vi "LIN_demo.vi"() -> ()   [LabVIEW 2020, in "zlgcan.lvlib"]
uses:
  zlgcan.lvlib
  ZCAN_LIN_MSG.ctl
  ZCAN_LIN_INIT_CONFIG_USBCANFD.ctl
  ZCAN_LIN_SUBSCIBE_CFG.ctl
  ZCAN_LIN_PUBLISH_CFG.ctl
  bin/zlgcan_wrap_LIN.dll
panel:
  in  "开启LIN":bool
  in  "?":T1(tab)
  in  "索引":u32(ring) items=["0", "1", "2", "3", "4", "5", "6", "7", "8"]
  in  "CAN卡型号":u32(ring)=41 items=["USBCANFD-400U"=76, "USBCANFD-800U"=59, "USBCANFD-200U"=41, "USBCANFD-100U"=42, "USBCANFD-MINI"=43]
  in  "LIN波特率（取值 1000~20000）":u32(ring)=9600 items=["19200"=19200, "9600"=9600, "4800"=4800, "2400"=2400]
  out "通道索引":u32(ring) items=["1"=1, "0"=0]
  in  "校验方式 （1-经典校验 2-增强校验 3-自动(即经典校验跟增强校验都会进行轮询)）":u8(ring)=1 items=["3"=3, "2"=2, "1"=1]
  out "LIN工作模式（从站为0，主站为1）":u8(ring) items=["1"=1, "0"=0]
  out "Device_handle(out)":u32
  out "lin1_index_handle(out)":u32
  out "lin0_index_handle(out)":u32
  in  "ID(hex)":u8=1 format="%x"
  in  "datalen":u8=8
  in  "数组长度":u32=1
  in  "chksumMode":u8=1
  in  "设置发布":bool
  in  "data十六进制hex":T2={"data[0]"=1, "data[1]"=2, "data[2]"=3, "data[3]"=4, "data[4]"=5, "data[5] "=6, "data[6] "=7, "data[7] "=8} {"data[7]" format="%x"; "data[6]" format="%x"; "data[5]" format="%x"; "data[0]" format="%x"; "data[1]" format="%x"; "data[2]" format="%x"; "data[3]" format="%x"; "data[4]" format="%x"}
  in  "设置订阅":bool
  in  "ID(Hex)":u8=1 format="%x"
  in  "datalen":u8=8
  in  "chkSumMode":u8=1
  in  "数组长度":u32=1
  in  "chnl 主站1":u8=1
  in  "dataType\n0为LIN数据":u8
  in  "ZCANLINData.PID(十六进制hex)":u8=1 format="%x"
  in  "datalen 数据长度":u8
  in  "timeStamp 时间戳 单位us":u64
  in  "dir 传输方向 0接收，1发送":u8
  in  "发送":bool
  out "已接收的帧数":u32
  out "LIN报文显示（仅显示LIN0从站的数据，方向针对的数据段而言）LIN类型为LIN错误数据则该数据出错，需要查看的话可自行二次开发":string[][](table)
  in  "LIN数据帧数组":T3[](array[typedef])
  in  "reserved":T4
  in  "ZCAN_LIN_PUBLISH_CFG":T5
  in  "reserved":T4
  in  "?":T6
  in  "chkSum 数据校验":u8
  in  "Reserved":u16
  in  "?":T7
  in  "ZCAN_LIN_MSG":T3
  in  "stop":bool
  in  "停止按钮":bool
  # "demo演示：LIN0通道做从站，LIN1通道做主站，仅主站可以往外发数据"
  # "流程：启动LIN----设置发布的ID等参数后，点击【设置发布】----LIN主站进行发送头部（PID跟发布的ID相同）"
  # "后面板已循环开启俩个LIN通道"
  # "1. 确保电脑有VC++ 2005/2008/2010/2013运行库（对应32，64位）,微软常用运行库合集，点击下载（35M）。\n    http://manual.zlg.cn/Public/Uploads/2020-06-05/5ed995c271414.zip"
  # "2，如果打开设备失败，可能原因：\n（1）已经打开过一次，没有正常关闭的情况下，继续点击“打开设备”，是无法打开的。\n     需要USB重新拔插，LABVIEW重启（全部关闭），然后再“打开设备”。\n (2) 项目路径不能有中文繁体。"
  # "LIN0(从站)设置发布，仅举例，可到后面板修改"
  # "用LIN1(主站)进行订阅数据"
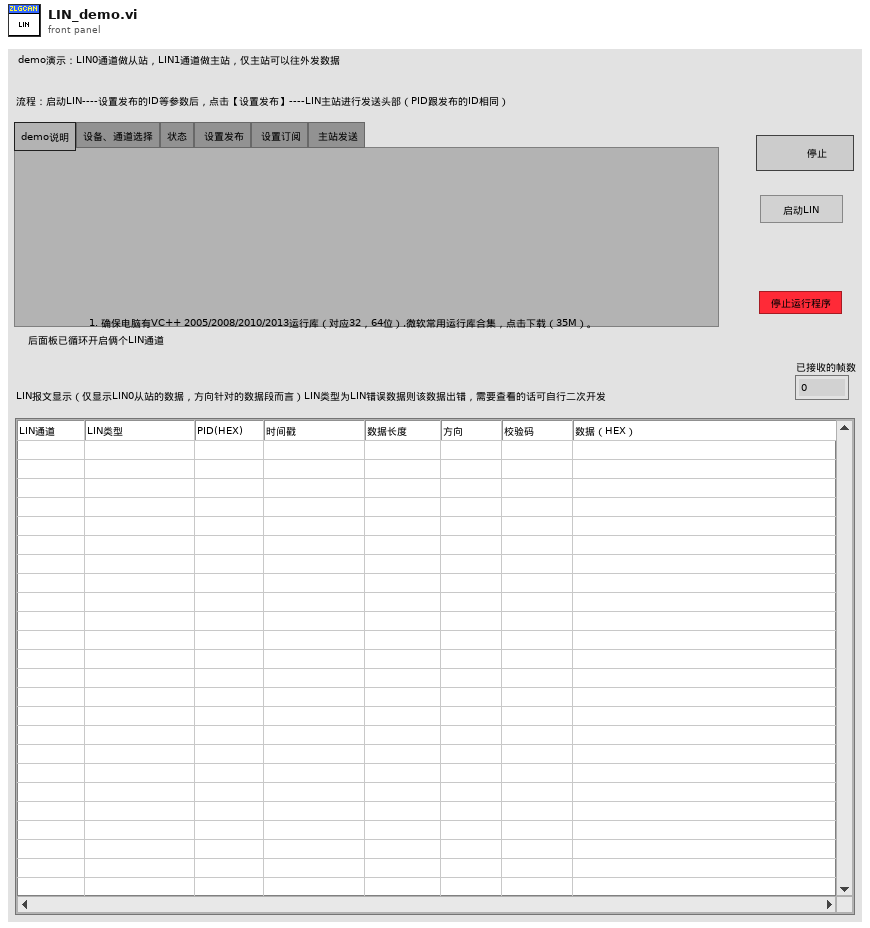
[diagram p1: front panel]
types:
  T1 = enum32{"demo说明", "设备、通道选择", "状态", " 设置发布", " 设置订阅", " 主站发送"}
  T2 = cluster{"data[0]":u8, "data[1]":u8, "data[2]":u8, "data[3]":u8, "data[4]":u8, "data[5] ":u8, "data[6] ":u8, "data[7] ":u8}
  T3 = typedef "zlgcan.lvlib/ZCAN_LIN_MSG.ctl" = cluster{"chnl":u8, "dataType":u8, "reserved 0":cluster{"CAN数据[0]":u8, "CAN数据[1]":u8, "CAN数据[2]":u8, "CAN数据[3]":u8, "CAN数据[4]":u8, "CAN数据[5]":u8}, "ZCANLINData":cluster{"PID":u8, "reserved":cluster{"CAN数据[0]":u8, "CAN数据[1]":u8, "CAN数据[2]":u8, "CAN数据[3]":u8, "CAN数据[4]":u8, "CAN数据[5]":u8, "CAN数据[6]":u8}, "RxData":cluster{"timeStamp":u64, "datalen":u8, "dir":u8, "chkSum":u8, "reserved[0]":u8, "reserved[1]":u8, "reserved[2] ":u8, "reserved[3]":u8, "reserved[4]":u8, "reserved[5]":u8, "reserved[6] ":u8, "reserved[7] ":u8, "reserved[8]":u8, "reserved[9] ":u8, "reserved[10] ":u8, "reserved[11] ":u8, "reserved[12] ":u8, "data[0]":u8, "data[1]":u8, "data[2]":u8, "data[3]":u8, "data[4]":u8, "data[5]":u8, "data[6]":u8, "data[7]":u8}}, "reserved 1":cluster{"CAN数据[0]":u8, "CAN数据[1]":u8, "CAN数据[2]":u8, "CAN数据[3]":u8, "CAN数据[4]":u8, "CAN数据[5]":u8}}
  T4 = cluster{"reserved[0]":u8, "reserved[1]":u8, "reserved[2]":u8, "reserved[3]":u8, "reserved[4]":u8}
  T5 = typedef "zlgcan.lvlib/ZCAN_LIN_PUBLISH_CFG.ctl" = cluster{"ID":u8, "datalen":u8, "data":cluster{"data[0]":u8, "data[1]":u8, "data[2]":u8, "data[3]":u8, "data[4]":u8, "data[5] ":u8, "data[6] ":u8, "data[7] ":u8}, "chkSumMode":u8, "reserved":cluster{"reserved[0]":u8, "reserved[1]":u8, "reserved[2]":u8, "reserved[3]":u8, "reserved[4]":u8}}
  T6 = typedef "zlgcan.lvlib/ZCAN_LIN_SUBSCIBE_CFG.ctl" = cluster{"ID":u8, "datalen":u8, "chkSumMode":u8, "reserved":cluster{"reserved[0]":u8, "reserved[1]":u8, "reserved[2]":u8, "reserved[3]":u8, "reserved[4]":u8}}
  T7 = typedef "zlgcan.lvlib/ZCAN_LIN_INIT_CONFIG_USBCANFD.ctl" = cluster{"LinMode":u8, "chkSumMode":u8, "Reserved":u16, "linBaud":u32}
  T8 = cluster{"CAN数据[0]":u8, "CAN数据[1]":u8, "CAN数据[2]":u8, "CAN数据[3]":u8, "CAN数据[4]":u8, "CAN数据[5]":u8}
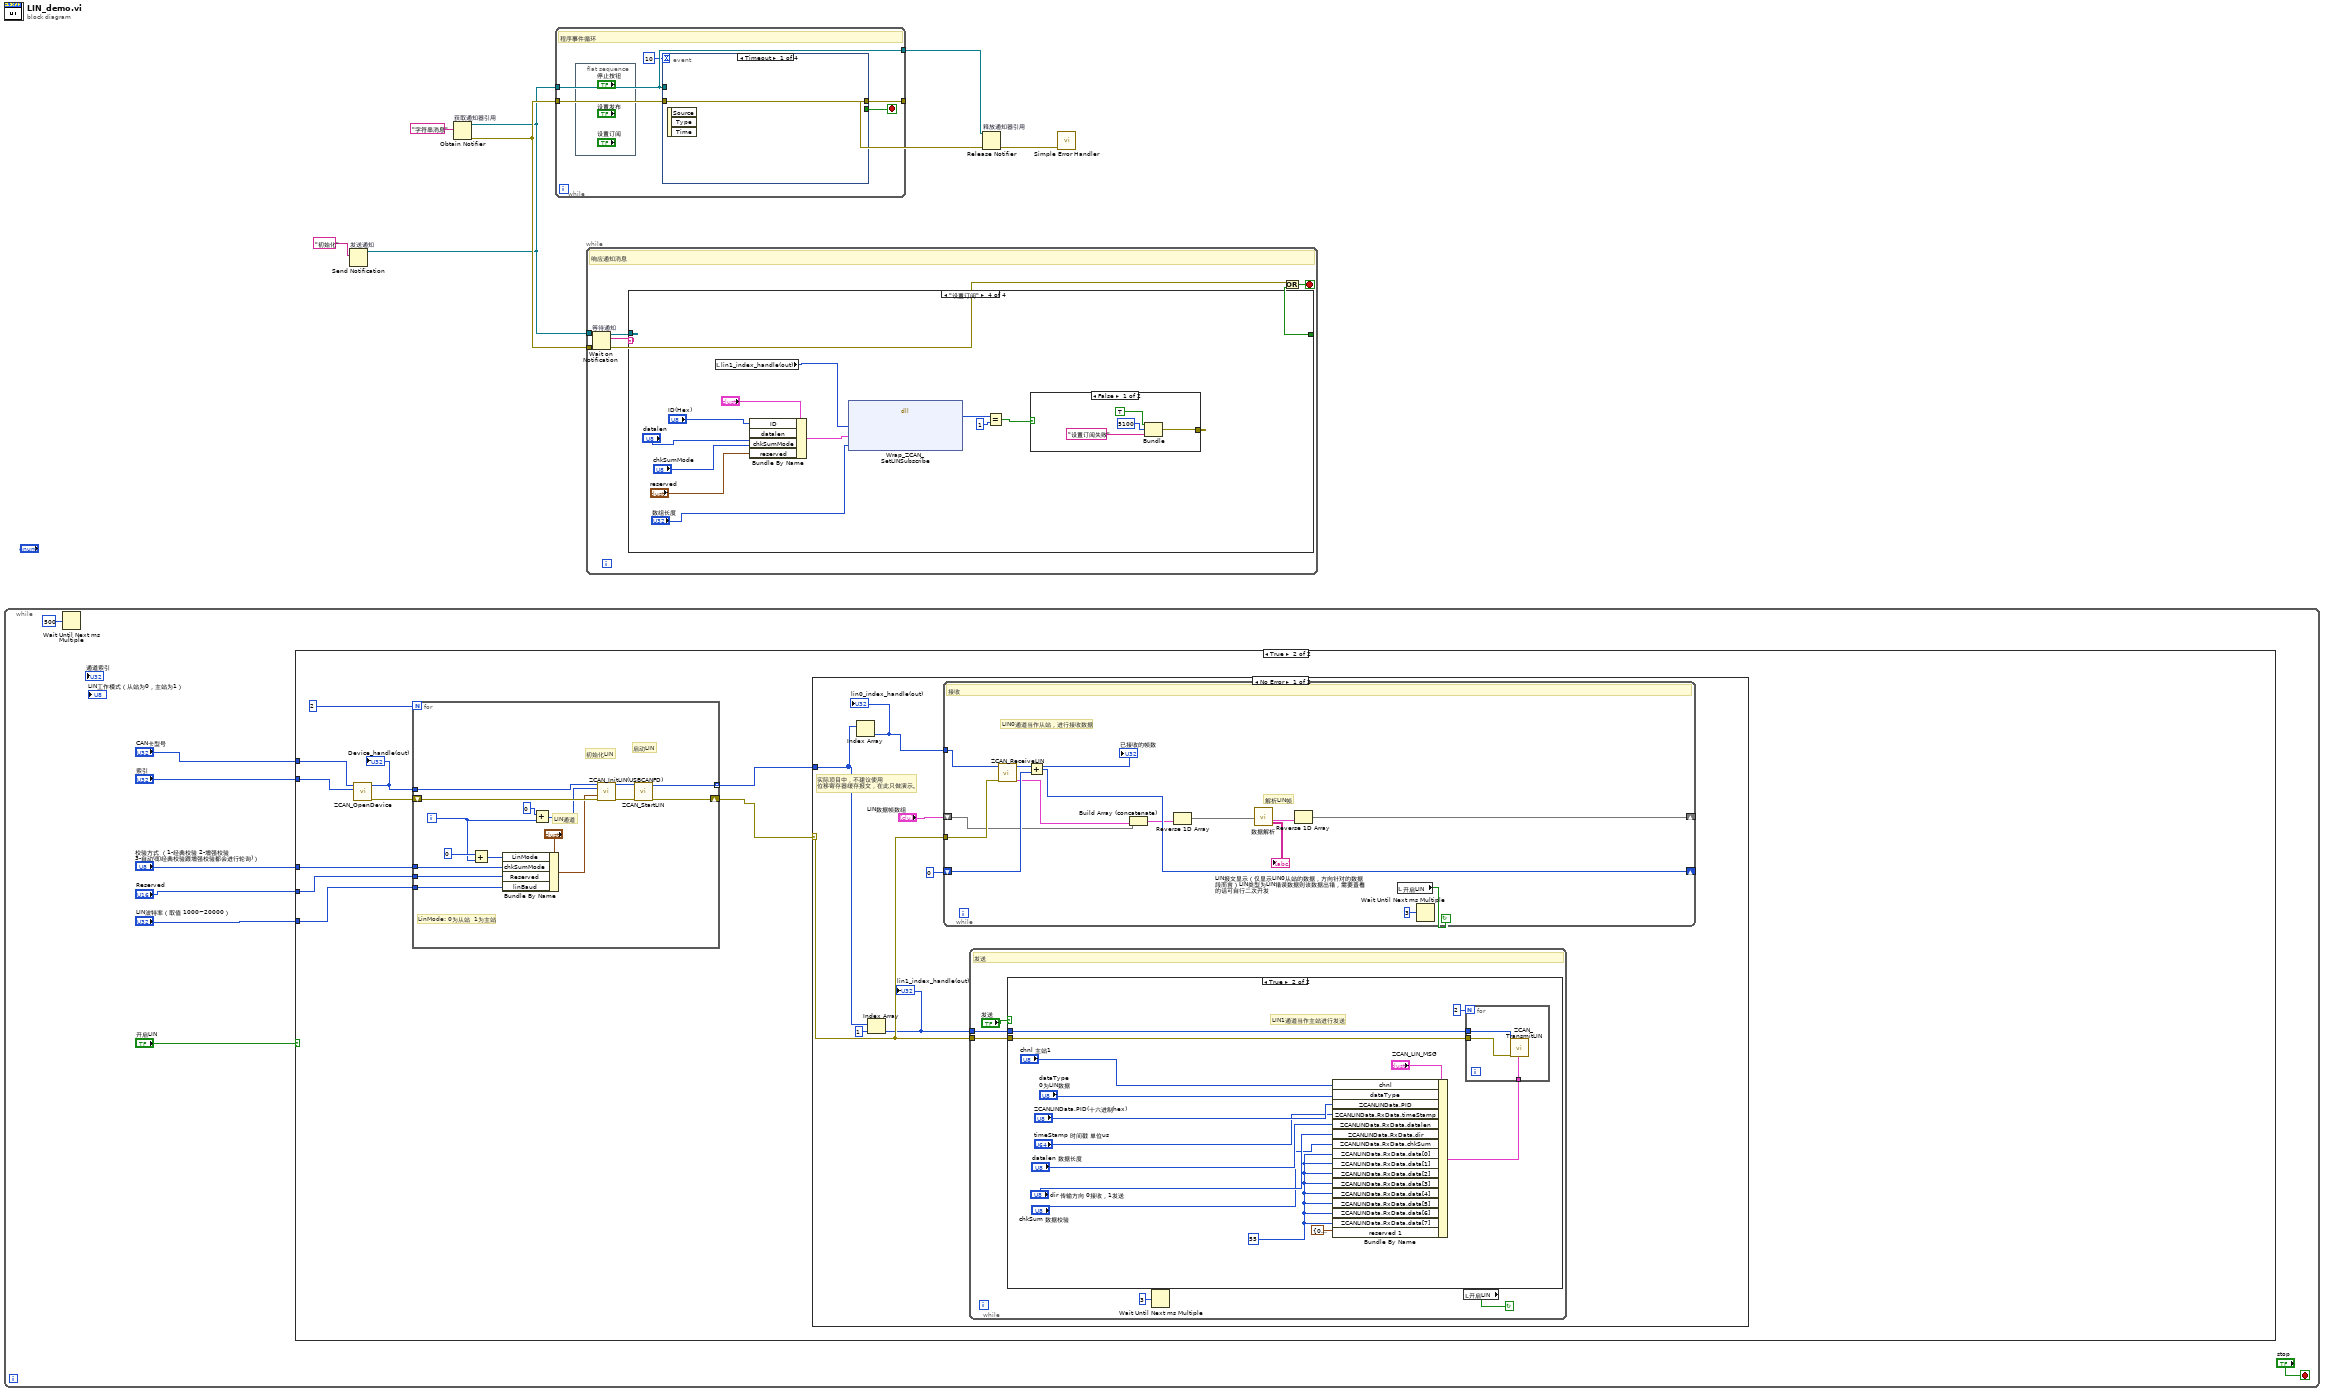
[diagram p0: block diagram]
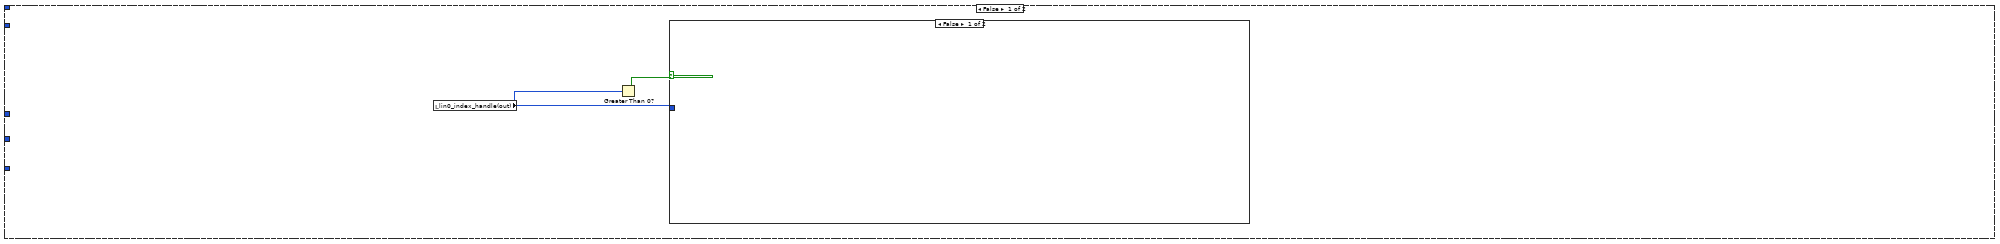
[diagram p2: hidden frame]
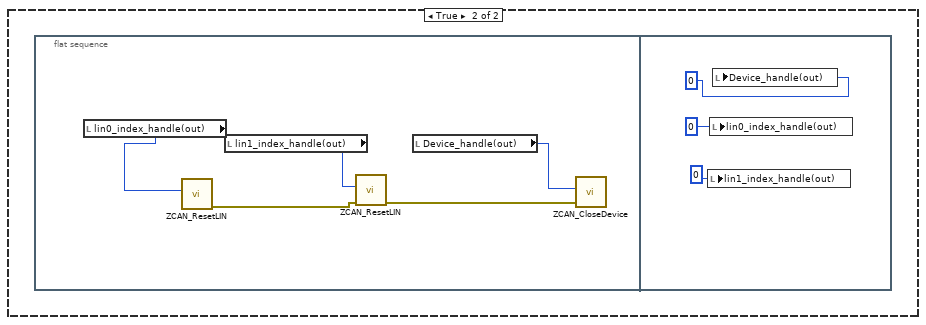
[diagram p3: hidden frame]
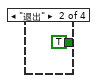
[diagram p7: hidden frame]
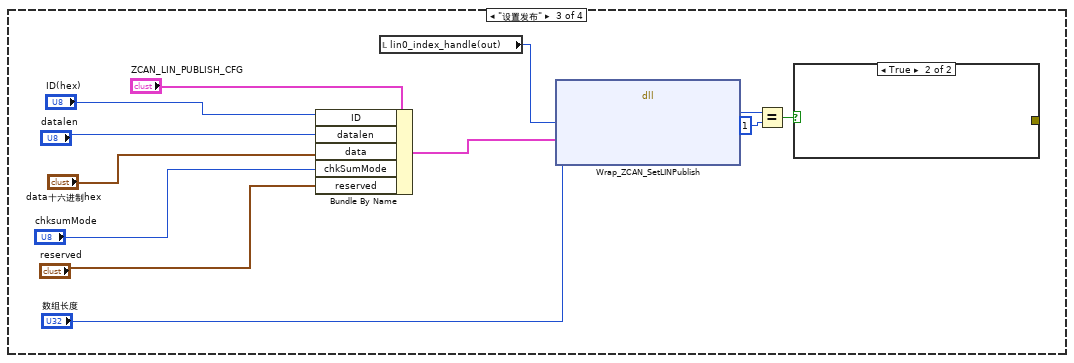
[diagram p8: hidden frame]
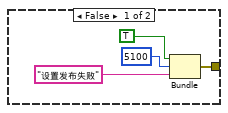
[diagram p9: hidden frame]
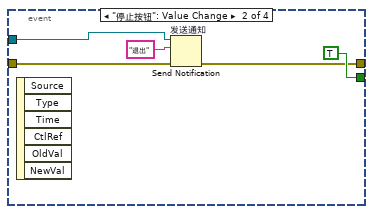
[diagram p11: hidden frame]
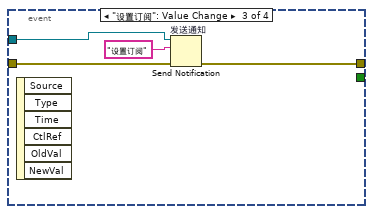
[diagram p12: hidden frame]
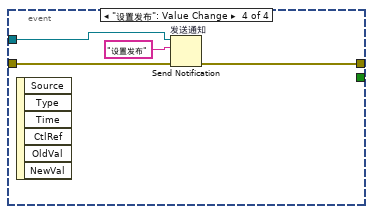
[diagram p13: hidden frame]
diagram:
  n1 = while {
    stop <- "stop" stop-if-true
    n2 = Wait Until Next ms Multiple(millisecond multiple=u32 500) -> ()  [unwired: 1 out]
    n3 = case shown="True" "开启LIN" {
      tunnel: "CAN卡型号" -> [_ w27]
      tunnel: "索引" -> [_ w26]
      tunnel: "LIN波特率（取值 1000~20000）" -> [_ w34]
      tunnel: "Reserved" -> [_ w33]
      tunnel: "校验方式 （1-经典校验 2-增强校验 3-自动(即经典校验跟增强校验都会进行轮询)）" -> [_ w31]
      frame False {
        # "关闭CAN卡"
        n4 = local read "lin0_index_handle(out)"() -> (w16:u32)
        n5 = Greater Than 0?(x=w16) -> (x > 0?=w17:bool)
        n6 = case shown="False" w17 {
          tunnel: w16 -> [_ _]
          frame False {
          }
          frame True {
            n7 = flat-sequence {
              frame #0 {
                n8 = local read "lin0_index_handle(out)"() -> (w22:u32)
                n9 = call "ZCAN_ResetLIN.vi"("lin_handle"=w22) -> ("error out"=w18:errorcluster)  [unwired: 9 in, 1 out]
                n10 = local read "lin1_index_handle(out)"() -> (w21:u32)
                n11 = call "ZCAN_ResetLIN.vi"("error in (no error)"=w18, "lin_handle"=w21) -> ("error out"=w20:errorcluster)  [unwired: 8 in, 1 out]
                n12 = local read "Device_handle(out)"() -> (w19:u32)
                n13 = call "ZCAN_CloseDevice.vi"("error in (no error)"=w20, "device_handle"=w19) -> ()  [unwired: 8 in, 2 out]
              }
              frame #1 {
                n14 = local write "lin1_index_handle(out)"(u32 0 ("lin1_index_handle(out)")) -> ()
                n15 = local write "lin0_index_handle(out)"(u32 0 ("lin0_index_handle(out)")) -> ()
                n16 = local write "Device_handle(out)"(u32 0 ("Device_handle(out)")) -> ()
              }
            }
          }
        }
      }
      frame True {
        n17 = call "ZCAN_OpenDevice.vi"("device_index"=w26, "device_type"=w27) -> ("error out"=w28:errorcluster, "DEVICE_HANDLE"=w29:u32)  [unwired: 6 in, 2 out]
        "Device_handle(out)" <- w29
        n18 = for {
          N: 2 -> [_]
          tunnel: [w36] -> w32 mode=indexing
          tunnel: w29 -> [w50]
          tunnel: w34 -> [w46]
          tunnel: w33 -> [w45]
          shift-right: [w49] -> w35
          shift-left: w28 -> [w51]
          tunnel: w31 -> [w39]
          i -> [w40]
          # "LinMode: 0为从站  1为主站"
          # "LIN通道"
          # "启动LIN"
          # "初始化LIN"
          n19 = Add(x=0, y=w40) -> (x+y=w41:i32)
          n20 = Bundle By Name(cluster="?", "LinMode"=w41, "chkSumMode"=w39, "Reserved"=w45, "linBaud"=w46) -> (w38:T7)
          n21 = Add(x=0, y=w40) -> (x+y=w44:i32)
          n22 = call "ZCAN_InitLIN(USBCANFD).vi"("device_hande"=w50, "lin_index"=w44, "ZCAN_LIN_INIT_CONFIG_USBCANFD"=w38, "error in (no error)"=w51) -> ("LIN_index_handle"=w37:u32, "error out"=w48:errorcluster)  [unwired: 10 in]
          n23 = call "ZCAN_StartLIN.vi"("error in (no error)"=w48, "lin_index_handle"=w37) -> ("error out"=w49:errorcluster, "lin_index_handle(out)"=w36:u32)  [unwired: 7 in, 1 out]
        }
        n24 = case shown="No Error" w35 {
          selector: w35 -> [w57 _]
          tunnel: w32 -> [w54 _]
          frame No Error {
            # "实际项目中，不建议使用\n位移寄存器缓存报文，在此只做演示。"
            n25 = Index Array(array=w54) -> (element=w53:u32)  [unwired: 1 in]
            "lin0_index_handle(out)" <- w53
            n26 = Index Array(array=w54, index=1 ("索引")) -> (element=w56:u32)
            "lin1_index_handle(out)" <- w56
            n27 = while {
              tunnel: w57 -> [w70]
              shift-right: [w71] -> _
              shift-left: 0 -> [w68]
              tunnel: w53 -> [w59]
              shift-right: [w60] -> _
              shift-left: "LIN数据帧数组" -> [w67]
              stop <- w69 continue-if-true
              # "解析LIN帧"
              # "LIN0通道当作从站，进行接收数据"
              # "接收"
              n28 = call "ZCAN_ReceiveLIN.vi"("error in (no error)"=w70, "channel_handle"=w59) -> ("LIN数据帧数组"=w62:T3[], "Receive_Num"=w66:u32)  [unwired: 4 in]
              "已接收的帧数" <- w66
              n29 = Add(x=w66, y=w68) -> (x+y=w71:u32)
              n30 = Build Array (concatenate)(w67, w62) -> (w65:T3[])
              n31 = Reverse 1D Array(array=w65) -> (reversed array=w64:T3[])
              n32 = call "数据解析.vi"("LIN数据帧数组"=w64) -> ("LIN数据帧数组 out"=w63:T3[], "LIN报文显示"=→"LIN报文显示（仅显示LIN0从站的数据，方向针对的数据段而言）LIN类型为LIN错误数据则该数据出错，需要查看的话可自行二次开发":string[][])  [unwired: 9 in]
              n33 = Reverse 1D Array(array=w63) -> (reversed array=w60:T3[])
              n34 = local read "开启LIN"() -> (w69:bool)
              n35 = Wait Until Next ms Multiple(millisecond multiple=u32 3) -> ()  [unwired: 1 out]
            }
            n36 = while {
              tunnel: w57 -> [w74]
              tunnel: w56 -> [w73]
              stop <- w75 continue-if-true
              # "发送"
              n37 = case shown="True" "发送" {
                tunnel: w74 -> [_ w89]
                tunnel: w73 -> [_ w90]
                frame False {
                }
                frame True {
                  w80 = u8 55 ("ZCANLINData.RxData.[data[0]")
                  # "LIN1通道当作主站进行发送"
                  n38 = Bundle By Name(cluster="ZCAN_LIN_MSG", "chnl"="chnl 主站1", "dataType"="dataType\n0为LIN数据", "ZCANLINData.PID"="ZCANLINData.PID(十六进制hex)", "ZCANLINData.RxData.timeStamp"="timeStamp 时间戳 单位us", "ZCANLINData.RxData.datalen"="datalen 数据长度", "ZCANLINData.RxData.dir"="dir 传输方向 0接收，1发送", "ZCANLINData.RxData.chkSum"="chkSum 数据校验", "ZCANLINData.RxData.data[0]"=w80, "ZCANLINData.RxData.data[1]"=w80, "ZCANLINData.RxData.data[2]"=w80, "ZCANLINData.RxData.data[3]"=w80, "ZCANLINData.RxData.data[4]"=w80, "ZCANLINData.RxData.data[5]"=w80, "ZCANLINData.RxData.data[6]"=w80, "ZCANLINData.RxData.data[7]"=w80, "reserved 1"=T8 {"CAN数据[0]"=0, "CAN数据[1]"=0, "CAN数据[2]"=0, "CAN数据[3]"=0, "CAN数据[4]"=0, "CAN数据[5]"=0}) -> (w88:T3)
                  n39 = for {
                    N: 2 -> [_]
                    tunnel: w90 -> [w94]
                    tunnel: w89 -> [w93]
                    tunnel: w88 -> [w92]
                    n40 = call "ZCAN_TransmitLIN.vi"("ZCAN_LIN_MSG"=w92, "error in (no error)"=w93, "lin_index_handle"=w94) -> ()  [unwired: 8 in, 1 out]
                  }
                }
              }
              n41 = Wait Until Next ms Multiple(millisecond multiple=u32 3) -> ()  [unwired: 1 out]
              n42 = local read "开启LIN"() -> (w75:bool)
            }
          }
          frame Error {
          }
        }
      }
    }
  }
  n43 = Obtain Notifier "获取通知器引用"(notification data type="字符串消息" ("元素数据类型")) -> (notifier out=w1:refnum<notifier>, error out=w6:errorcluster)  [unwired: 3 in, 1 out]
  n44 = Send Notification "发送通知"(notification="初始化" ("通知"), notifier=w1) -> ()  [unwired: 1 in, 2 out]
  n45 = while "While循环" {
    tunnel: w1 -> [w96]
    tunnel: [w96] -> w7
    tunnel: w6 -> [w98]
    tunnel: [w97] -> w5
    stop <- w99 stop-if-true
    # "程序事件循环"
    n46 = flat-sequence {
      frame #0 {
      }
    }
    n47 = event shown="[0] Timeout" {
      selector: _ -> [_ _ _ _]
      dyn-events: _ -> [_ _ _ _]
      timeout: 10 -> [_ _ _ _]
      tunnel: w96 -> [_ w103 w108 w112]
      tunnel: [_ TRUE _ _] -> w99
      tunnel: w98 -> [w100 w102 w107 w111]
      tunnel: [w100 w101 w106 w110] -> w97
      event Timeout {
        n48 = event-data() -> ()  [unwired: 1 in, 3 out]
      }
      event "停止按钮": Value Change {
        n49 = event-data() -> ()  [unwired: 1 in, 6 out]
        n50 = Send Notification "发送通知"(notification="退出" ("通知"), notifier=w103, error in (no error)=w102) -> (error out=w101:errorcluster)  [unwired: 1 out]
      }
      event "设置订阅": Value Change {
        n51 = event-data() -> ()  [unwired: 1 in, 6 out]
        n52 = Send Notification "发送通知"(notification="设置订阅" ("通知"), notifier=w108, error in (no error)=w107) -> (error out=w106:errorcluster)  [unwired: 1 out]
      }
      event "设置发布": Value Change {
        n53 = event-data() -> ()  [unwired: 1 in, 6 out]
        n54 = Send Notification "发送通知"(notification="设置发布" ("通知"), notifier=w112, error in (no error)=w111) -> (error out=w110:errorcluster)  [unwired: 1 out]
      }
    }
  }
  n55 = while "While循环" {
    tunnel: w1 -> [w120]
    tunnel: w6 -> [w118]
    stop <- w117 stop-if-true
    # "响应通知消息"
    n56 = Wait on Notification "等待通知"(notifier=w120, error in (no error)=w118) -> (notifier out=w116:refnum<notifier>, notification=w119:string, error out=w115:errorcluster)  [unwired: 2 in, 1 out]
    n57 = case shown="\"设置订阅\"" w119 {
      tunnel: [_ TRUE _ _] -> w114
      tunnel: w116 -> [_ _ _ _]
      frame Default {
      }
      frame "退出" {
      }
      frame "设置发布" {
        n58 = Bundle By Name(cluster="ZCAN_LIN_PUBLISH_CFG", "ID"="ID(hex)", "datalen"="datalen", "data"="data十六进制hex", "chkSumMode"="chksumMode", "reserved"="reserved") -> (w129:T5)
        n59 = local read "lin0_index_handle(out)"() -> (w122:u32)
        n60 = dll-call lib="D:/Git/ZLG_USBCANFD/bin/zlgcan_wrap_LIN.dll" fn="Wrap_ZCAN_SetLINPublish"("通道句柄"=w122, "ZCAN_LIN_PUBLISH_CFG"=w129, "数组长度"="数组长度") -> ("返回类型"=w133:u32)  [unwired: 6 in, 2 out]
        n61 = Equal?(x=w133, y=u32 1) -> (x = y?=w132:bool)
        n62 = case shown="True" w132 {
          tunnel: [w134 _] -> _
          frame False {
            n63 = Bundle("status"=TRUE, "code"=5100, "消息"="设置发布失败") -> (w134:cluster{"status":bool, "code":i32, "消息":string})  [unwired: 1 in]
          }
          frame True {
          }
        }
      }
      frame "设置订阅" {
        n64 = local read "lin1_index_handle(out)"() -> (w138:u32)
        n65 = Bundle By Name(cluster="?", "ID"="ID(Hex)", "datalen"="datalen", "chkSumMode"="chkSumMode", "reserved"="reserved") -> (w145:T6)
        n66 = dll-call lib="D:/Git/ZLG_USBCANFD/bin/zlgcan_wrap_LIN.dll" fn="Wrap_ZCAN_SetLINSubscribe"("通道句柄"=w138, "ZCAN_LIN_SUBSCIBE_CFG"=w145, "数组长度"="数组长度") -> ("返回类型"=w148:u32)  [unwired: 6 in, 2 out]
        n67 = Equal?(x=w148, y=u32 1) -> (x = y?=w147:bool)
        n68 = case shown="False" w147 {
          tunnel: [w149 _] -> _
          frame False {
            n69 = Bundle("status"=TRUE, "code"=5100, "消息"="设置订阅失败") -> (w149:cluster{"status":bool, "code":i32, "消息":string})  [unwired: 1 in]
          }
          frame True {
          }
        }
      }
    }
    n70 = Or(x=w115, y=w114) -> (x .or. y?=w117:bool)
  }
  n71 = Release Notifier "释放通知器引用"(notifier=w7, error in (no error)=w5) -> (error out=w4:errorcluster)  [unwired: 1 in, 2 out]
  n72 = call <vilib>:"Simple Error Handler.vi"("error in (no error)"=w4) -> ()  [unwired: 4 in, 5 out]
